vi "MC.SetWavelength.vi"(8 "error in (no error)":errorcluster, 10 "Wavelength, nm":dbl=620.0, 11 "MC.DangwooOptron":refnum<class "MC.DangwooOptron.lvclass">) -> (0 "error out":errorcluster, 3 "MC.DangwooOptron out":refnum<class "MC.DangwooOptron.lvclass">)   [LabVIEW 2017, in "MC.DangwooOptron.lvclass"]
doc: "---------------------------------------------------------------\nJKI State Machine Objects™\nhttp://jki.net/state-machine-objects/\nCopyright (C) 2005-2015, JKI <info@jki.net>\nALL RIGHTS RESERVEDJKI State Machine Objects (SMO) 1.0.0.5\nJKI - JKI\nCopyright (c) 2016, JKI"
uses:
  MC.DangwooOptron.lvclass
panel:
  out "read buffer":string
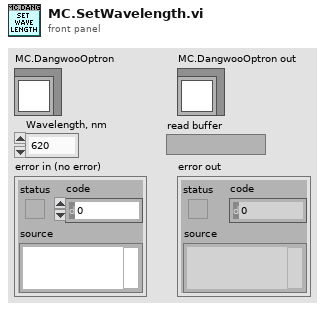
[diagram p1: front panel]
types:
  T1 = typedef "MC.DangwooOptron.lvclass/Resource--Cluster.ctl" = cluster{"VISA resource":refnum<visa-resource-name>}
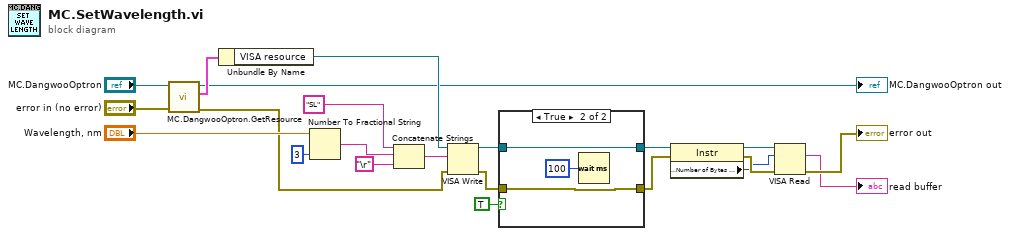
[diagram p0: block diagram]
diagram:
  n1 = call "MC.DangwooOptron.GetResource.vi"("error in (no error)"="error in (no error)", "MC.DangwooOptron"="MC.DangwooOptron") -> ("error out"=w12:errorcluster, "Resource"=w14:T1, "MC.DangwooOptron out"=→"MC.DangwooOptron out":refnum<class "MC.DangwooOptron.lvclass">)  [unwired: 7 in]
  n2 = Unbundle By Name(w14) -> ("VISA resource"=w13:refnum<visa-resource-name>)
  n3 = Number To Fractional String(number="Wavelength, nm", precision (6)=3) -> (F-format string=w18:string)  [unwired: 2 in]
  n4 = Concatenate Strings("SL" ("SL"), w18, "\r") -> (w20:string)
  n5 = VISA Write(VISA resource name=w13, write buffer=w20, error in (no error)=w12) -> (VISA resource name out=w9:refnum<visa-resource-name>, error out=w8:errorcluster)  [unwired: 1 out]
  n6 = case shown="True" TRUE {
    tunnel: [w24 w26] -> w7
    tunnel: w9 -> [w24 w26]
    tunnel: w8 -> [w23 w25]
    tunnel: [w23 w25] -> w6
    frame False {
    }
    frame True {
      n7 = Wait (ms)(milliseconds to wait=u32 100) -> ()  [unwired: 1 out]
    }
  }
  n8 = property class="Instr"(reference=w7, error in=w6) -> (reference out=w5:refnum<visa-resource-name>, error out=w4:errorcluster, "Serial Settings:Number of Bytes at Serial Port"=w3:u32)
  n9 = VISA Read(VISA resource name=w5, byte count=w3, error in (no error)=w4) -> (read buffer=→"read buffer":string, error out=→"error out":errorcluster)  [unwired: 2 out]
